vi "AVS_Read_Ch6+7.vi"() -> (0 "Resistance reading ch 6":dbl format="%.2f", 1 "Resistance reading ch 5":dbl format="%.2f", 2 "Resistance reading ch 7":dbl format="%.2f")   [LabVIEW 2018]
uses:
  Instrument_Setup_v2.vi
  data/Data_Display_global.vi
panel:
  out "T (K) ch7":dbl=0.00957168277075326 format="%^.3e"
  out "T (K) ch6":dbl=0.00957168277075326 format="%^.3e"
  out "T (K) ch5":dbl=0.00957168277075326 format="%^.3e"
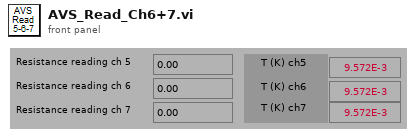
[diagram p1: front panel]
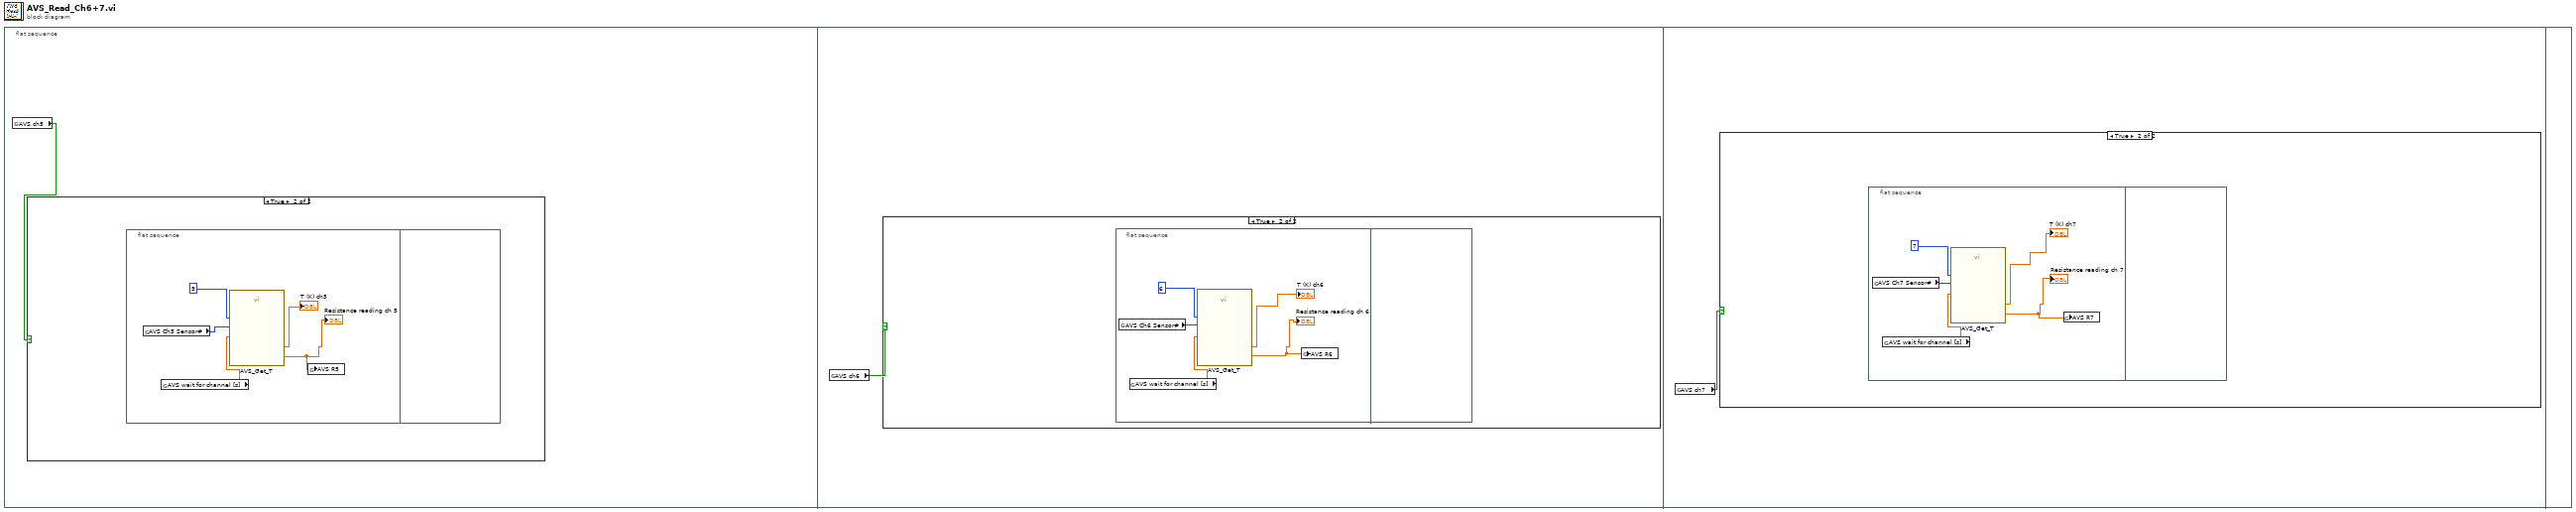
[diagram p0: block diagram]
diagram:
  n1 = flat-sequence {
    frame #0 {
      n2 = global read "Instrument_Setup_v2.vi" "AVS ch5"() -> (w1:bool)
      n3 = case shown="True" w1 {
        frame False {
        }
        frame True {
          n4 = flat-sequence {
            frame #0 {
              n5 = global read "Instrument_Setup_v2.vi" "AVS Ch5 Sensor#"() -> (w3:u16)
              n6 = global read "Instrument_Setup_v2.vi" "AVS wait for channel [s]"() -> (w4:dbl)
              n7 = call "AVS_Get_T.vi"("Sensor Calib"=w3, "AVS Channel"=i8 5 ("CHANNEL (-1:no change )"), "Wait for channel (s)"=w4) -> ("Resistance reading"=w2:dbl, "T (K)"=→"T (K) ch5":dbl)  [unwired: 7 in]
              "Resistance reading ch 5" <- w2
              n8 = global write "Data_Display_global.vi" "AVS R5"(w2) -> ()
            }
            frame #1 {
            }
          }
        }
      }
    }
    frame #1 {
      n9 = global read "Instrument_Setup_v2.vi" "AVS ch6"() -> (w7:bool)
      n10 = case shown="True" w7 {
        frame False {
        }
        frame True {
          n11 = flat-sequence {
            frame #0 {
              n12 = global read "Instrument_Setup_v2.vi" "AVS Ch6 Sensor#"() -> (w9:u16)
              n13 = global read "Instrument_Setup_v2.vi" "AVS wait for channel [s]"() -> (w11:dbl)
              n14 = call "AVS_Get_T.vi"("Sensor Calib"=w9, "AVS Channel"=i8 6 ("CHANNEL (-1:no change )"), "Wait for channel (s)"=w11) -> ("Resistance reading"=w8:dbl, "T (K)"=→"T (K) ch6":dbl)  [unwired: 7 in]
              "Resistance reading ch 6" <- w8
              n15 = global write "Data_Display_global.vi" "AVS R6"(w8) -> ()
            }
            frame #1 {
            }
          }
        }
      }
    }
    frame #2 {
      n16 = global read "Instrument_Setup_v2.vi" "AVS ch7"() -> (w13:bool)
      n17 = case shown="True" w13 {
        frame False {
        }
        frame True {
          n18 = flat-sequence {
            frame #0 {
              n19 = global read "Instrument_Setup_v2.vi" "AVS Ch7 Sensor#"() -> (w16:u16)
              n20 = global read "Instrument_Setup_v2.vi" "AVS wait for channel [s]"() -> (w17:dbl)
              n21 = call "AVS_Get_T.vi"("Sensor Calib"=w16, "AVS Channel"=i8 7 ("CHANNEL (-1:no change )"), "Wait for channel (s)"=w17) -> ("Resistance reading"=w14:dbl, "T (K)"=→"T (K) ch7":dbl)  [unwired: 7 in]
              "Resistance reading ch 7" <- w14
              n22 = global write "Data_Display_global.vi" "AVS R7"(w14) -> ()
            }
            frame #1 {
            }
          }
        }
      }
    }
    frame #3 {
    }
  }
